vi "Decode Balls.vi"(5 "Time Stamp":timestamp, 8 "error in":errorcluster, 9 "array":u8[](array[numeric]), 10 "Key":i32=5) -> (0 "error out":errorcluster, 1 "array w/ subset deleted out":u8[](array[numeric]), 3 "Array":T1[](array[typedef]))   [LabVIEW 2017]
uses:
  SSL Detection Ball.ctl
  <vilib>/Analysis/Matrix/Datatypes/RealMatrix.ctl
  <vilib>/Analysis/Matrix/NI_Matrix.lvlib
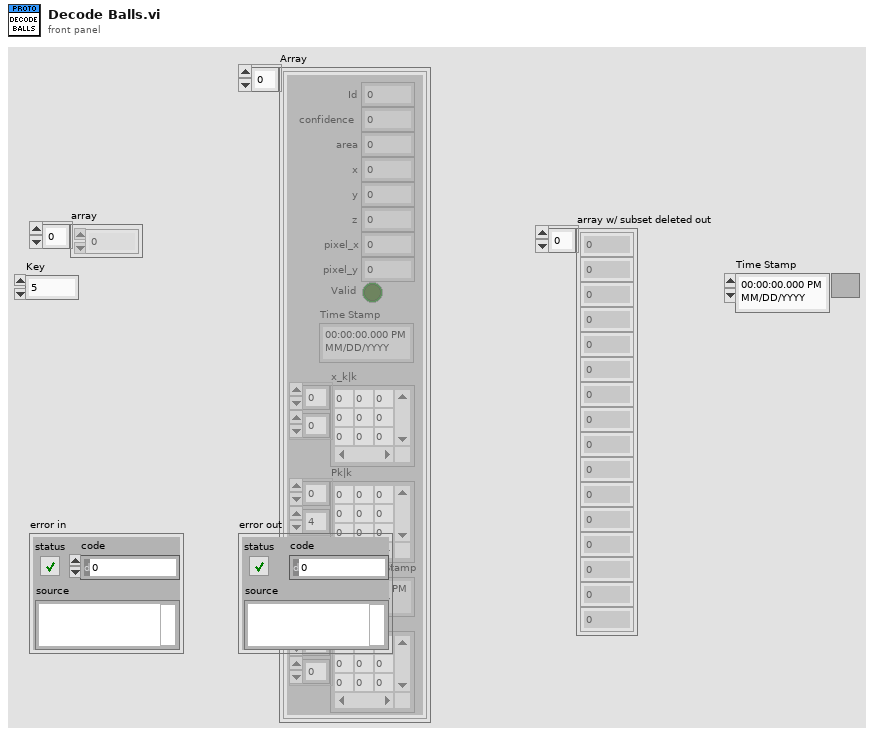
[diagram p1: front panel]
types:
  T1 = typedef "SSL Detection Ball.ctl" = cluster{"x":sgl, "area":u32, "confidence":sgl, "y":sgl, "z":sgl, "pixel_x":sgl, "pixel_y":sgl, "Valid":bool, "Time Stamp":timestamp, "x_k|k":T2, "Pk|k":T2, "Id":u32, "Previous Time Stamp":timestamp, "R":T2}
  T2 = typedef "NI_Matrix.lvlib/RealMatrix.ctl" = dbl[][]
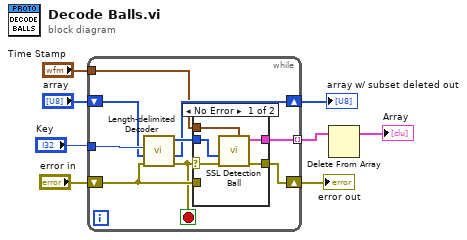
[diagram p0: block diagram]
diagram:
  n1 = while {
    shift-right: [w14] -> w5
    shift-left: "array" -> [w10]
    tunnel: [w17] -> w4 mode=indexing
    shift-right: [w16] -> w7
    shift-left: "error in" -> [w13]
    tunnel: "Key" -> [w11]
    tunnel: "Time Stamp" -> [w9]
    stop <- w12 stop-if-true
    n2 = call "Length-delimited Decoder.vi"("error in (no error)"=w13, "Array"=w10, "Key"=w11) -> ("error out"=w12:errorcluster, "array w/ subset deleted"=w14:u8[], "Length-delimited"=w15:u8[])  [unwired: 5 in, 1 out]
    n3 = case shown="No Error" w12 {
      selector: w12 -> [w20 _]
      tunnel: [w22 _] -> w17
      tunnel: [w21 w23] -> w16
      tunnel: w15 -> [w19 _]
      tunnel: w13 -> [_ w23]
      tunnel: w9 -> [w18 _]
      frame No Error {
        n4 = call "SSL Detection Ball.vi"("Time Stamp"=w18, "error in"=w20, "Array"=w19) -> ("error out"=w21:errorcluster, "Detection Ball"=w22:T1)  [unwired: 6 in, 1 out]
      }
      frame Error {
      }
    }
  }
  "error out" <- w7
  "array w/ subset deleted out" <- w5
  n5 = Delete From Array(array=w4) -> (array with subset deleted=→"Array":T1[])  [unwired: 2 in, 1 out]
